vi "Analog Input User Interface.vi"() -> ()   [LabVIEW 2023, in "GUI.lvlib" / "Diagnostic.lvlib"]
uses:
  Diagnostic.lvlib
  Control/Analog Input 6345.ctl
  Control/Analog Input.ctl
  Control/Analog Input 6363.ctl
  HardwareAbstractionLayer_LVOOP/Analog Input/NI Analog Input/NI Analog Input.lvclass
  D:/eDCU LTT/VT LTT Project/Source Code/HardwareAbstractionLayer_LVOOP/Analog Input/AI/AI.lvclass
  HardwareAbstractionLayer_LVOOP/Database/SQL Public VI/Control/DB Options.ctl
  HardwareAbstractionLayer_LVOOP/Main/Class Ref.ctl
  HardwareAbstractionLayer_LVOOP/DMM/DMM.lvclass
  HardwareAbstractionLayer_LVOOP/Function Generator/Function Generator.lvclass
  HardwareAbstractionLayer_LVOOP/Oscilloscope/Oscilloscope.lvclass
  HardwareAbstractionLayer_LVOOP/PowerSupply/PowerSupply.lvclass
  HardwareAbstractionLayer_LVOOP/Teststand/Teststand.lvclass
  HardwareAbstractionLayer_LVOOP/Analog Output/AO/AO.lvclass
  HardwareAbstractionLayer_LVOOP/Analog Input/AI/AI.lvclass
  HardwareAbstractionLayer_LVOOP/Database/Database.lvclass
  HardwareAbstractionLayer_LVOOP/Digital Output/DO_class/DO.lvclass
  HardwareAbstractionLayer_LVOOP/Digital Input/DI_class/DI.lvclass
  HardwareAbstractionLayer_LVOOP/PWM Output/PWM Output_class/PWM Output.lvclass
  HardwareAbstractionLayer_LVOOP/PWM Input/PWM Input_class/PWM Input.lvclass
  HardwareAbstractionLayer_LVOOP/NI Switch/NISwitch_class/NISwitch.lvclass
  HardwareAbstractionLayer_LVOOP/Modbus/Modbus_class/Modbus.lvclass
  HardwareAbstractionLayer_LVOOP/CAN/CAN Lib/CAN_class/CAN.lvclass
  HardwareAbstractionLayer_LVOOP/Main/Main.lvclass
panel:
  in  "Stop Acquire":bool
  in  "Start Acquire":bool
  out "error out":errorcluster
  in  "error in":errorcluster
  in  "Operation":enum32{"6345-PXI2Slot3", "6363-PXI2Slot2"}(tab)
  out "PXIe - 6345":T1 {"Channel 31" format="%.3g"; "Channel 30" format="%.3g"; "Channel 29" format="%.3g"; "Channel 28" format="%.3g"; "Channel 27" format="%.3g"; "Channel 26" format="%.3g"; "Channel 25" format="%.3g"; "Channel 24" format="%.3g"; "Channel 23" format="%.3g"; "Channel 22" format="%.3g"; "Channel 21" format="%.3g"; "Channel 20" format="%.3g"; "Channel 19" format="%.3g"; "Channel 18" format="%.3g"; "Channel 17" format="%.3g"; "Channel 16" format="%.3g"; "Channel 79" format="%.3g"; "Channel 78" format="%.3g"; "Channel 77" format="%.3g"; "Channel 76" format="%.3g"; "Channel 75" format="%.3g"; "Channel 74" format="%.3g"; "Channel 73" format="%.3g"; "Channel 72" format="%.3g"; "Channel 71" format="%.3g"; "Channel 70" format="%.3g"; "Channel 69" format="%.3g"; "Channel 68" format="%.3g"; "Channel 67" format="%.3g"; "Channel 66" format="%.3g"; "Channel 65" format="%.3g"; "Channel 64" format="%.3g"; "Channel 63" format="%.3g"; "Channel 62" format="%.3g"; "Channel 61" format="%.3g"; "Channel 60" format="%.3g"; "Channel 59" format="%.3g"; "Channel 58" format="%.3g"; "Channel 57" format="%.3g"; "Channel 56" format="%.3g"; "Channel 55" format="%.3g"; "Channel 54" format="%.3g"; "Channel 53" format="%.3g"; "Channel 52" format="%.3g"; "Channel 51" format="%.3g"; "Channel 50" format="%.3g"; "Channel 49" format="%.3g"; "Channel 48" format="%.3g"; "Channel 47" format="%.3g"; "Channel 46" format="%.3g"; "Channel 45" format="%.3g"; "Channel 44" format="%.3g"; "Channel 43" format="%.3g"; "Channel 42" format="%.3g"; "Channel 41" format="%.3g"; "Channel 40" format="%.3g"; "Channel 39" format="%.3g"; "Channel 38" format="%.3g"; "Channel 37" format="%.3g"; "Channel 36" format="%.3g"; "Channel 35" format="%.3g"; "Channel 34" format="%.3g"; "Channel 33" format="%.3g"; "Channel 32" format="%.3g"; "Channel 15" format="%.3g"; "Channel 14" format="%.3g"; "Channel 13" format="%.3g"; "Channel 12" format="%.3g"; "Channel 11" format="%.3g"; "Channel 10" format="%.3g"; "Channel 9" format="%.3g"; "Channel 8" format="%.3g"; "Channel 7" format="%.3g"; "Channel 6" format="%.3g"; "Channel 5" format="%.3g"; "Channel 4" format="%.3g"; "Channel 3" format="%.3g"; "Channel 2" format="%.3g"; "Channel 1" format="%.3g"; "Channel 0" format="%.3g"}
  out "PXIe - 6363":T3 {"Channel 31" format="%.3g"; "Channel 30" format="%.3g"; "Channel 29" format="%.3g"; "Channel 28" format="%.3g"; "Channel 27" format="%.3g"; "Channel 26" format="%.3g"; "Channel 25" format="%.3g"; "Channel 24" format="%.3g"; "Channel 23" format="%.3g"; "Channel 22" format="%.3g"; "Channel 21" format="%.3g"; "Channel 20" format="%.3g"; "Channel 19" format="%.3g"; "Channel 18" format="%.3g"; "Channel 17" format="%.3g"; "Channel 16" format="%.3g"; "Channel 15" format="%.3g"; "Channel 14" format="%.3g"; "Channel 13" format="%.3g"; "Channel 12" format="%.3g"; "Channel 11" format="%.3g"; "Channel 10" format="%.3g"; "Channel 9" format="%.3g"; "Channel 8" format="%.3g"; "Channel 7" format="%.3g"; "Channel 6" format="%.3g"; "Channel 5" format="%.3g"; "Channel 4" format="%.3g"; "Channel 3" format="%.3g"; "Channel 2" format="%.3g"; "Channel 1" format="%.3g"; "Channel 0" format="%.3g"}
  in  "Stop":bool caption="Blank"
  # "Analog Input"
  # "Device:"
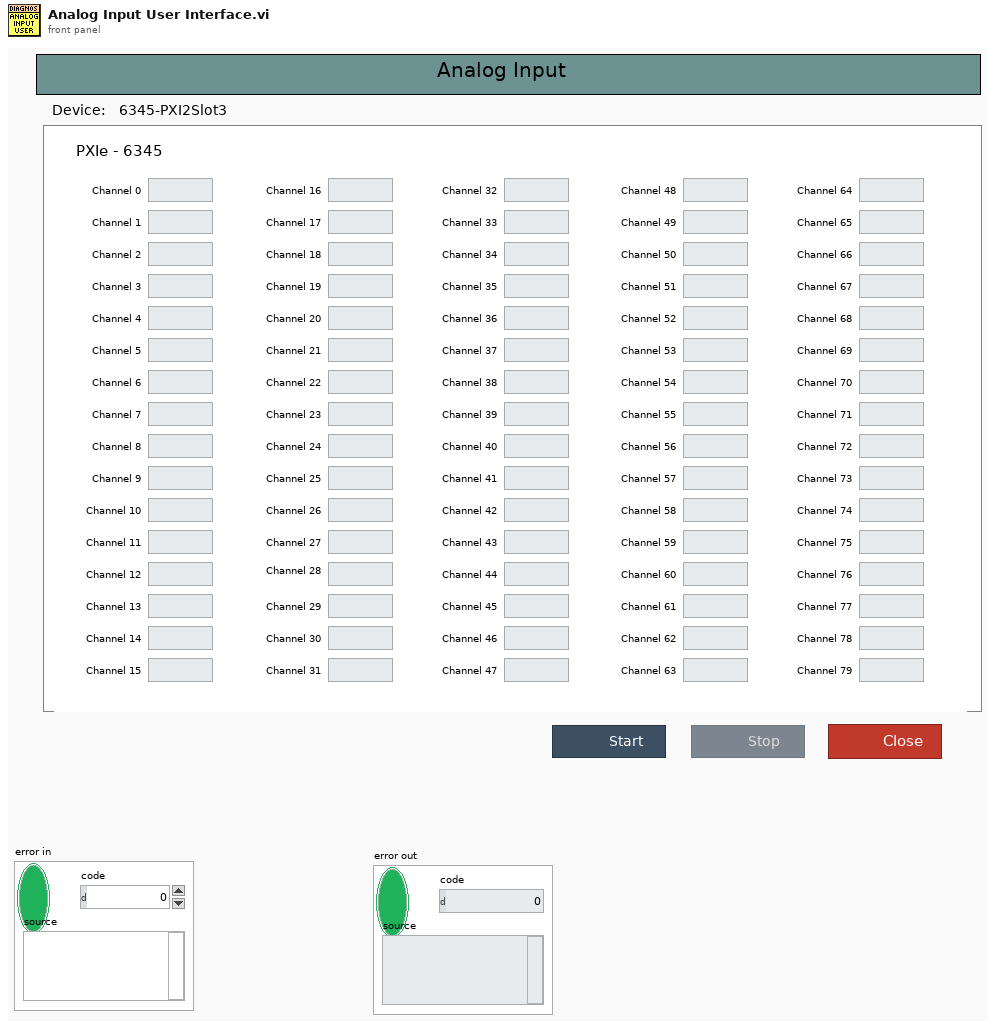
[diagram p1: front panel]
types:
  T1 = typedef "GUI.lvlib/Diagnostic.lvlib/Analog Input 6345.ctl" = cluster{"Channel 0":T2, "Channel 1":T2, "Channel 2":T2, "Channel 3":T2, "Channel 4":T2, "Channel 5":T2, "Channel 6":T2, "Channel 7":T2, "Channel 8":T2, "Channel 9":T2, "Channel 10":T2, "Channel 11":T2, "Channel 12":T2, "Channel 13":T2, "Channel 14":T2, "Channel 15":T2, "Channel 16":T2, "Channel 17":T2, "Channel 18":T2, "Channel 19":T2, "Channel 20":T2, "Channel 21":T2, "Channel 22":T2, "Channel 23":T2, "Channel 24":T2, "Channel 25":T2, "Channel 26":T2, "Channel 27":T2, "Channel 28":T2, "Channel 29":T2, "Channel 30":T2, "Channel 32":T2, "Channel 33":T2, "Channel 34":T2, "Channel 35":T2, "Channel 36":T2, "Channel 37":T2, "Channel 38":T2, "Channel 39":T2, "Channel 40":T2, "Channel 41":T2, "Channel 42":T2, "Channel 43":T2, "Channel 44":T2, "Channel 45":T2, "Channel 46":T2, "Channel 47":T2, "Channel 48":T2, "Channel 49":T2, "Channel 50":T2, "Channel 51":T2, "Channel 52":T2, "Channel 53":T2, "Channel 54":T2, "Channel 55":T2, "Channel 56":T2, "Channel 57":T2, "Channel 58":T2, "Channel 59":T2, "Channel 60":T2, "Channel 61":T2, "Channel 62":T2, "Channel 63":T2, "Channel 64":T2, "Channel 65":T2, "Channel 66":T2, "Channel 67":T2, "Channel 68":T2, "Channel 69":T2, "Channel 70":T2, "Channel 71":T2, "Channel 72":T2, "Channel 73":T2, "Channel 74":T2, "Channel 75":T2, "Channel 76":T2, "Channel 77":T2, "Channel 78":T2, "Channel 79":T2, "Channel 31":T2}
  T2 = typedef "GUI.lvlib/Diagnostic.lvlib/Analog Input.ctl" = dbl
  T3 = typedef "GUI.lvlib/Diagnostic.lvlib/Analog Input 6363.ctl" = cluster{"Channel 0":T2, "Channel 1":T2, "Channel 2":T2, "Channel 3":T2, "Channel 4":T2, "Channel 5":T2, "Channel 6":T2, "Channel 7":T2, "Channel 8":T2, "Channel 9":T2, "Channel 10":T2, "Channel 11":T2, "Channel 12":T2, "Channel 13":T2, "Channel 14":T2, "Channel 15":T2, "Channel 16":T2, "Channel 17":T2, "Channel 18":T2, "Channel 19":T2, "Channel 20":T2, "Channel 21":T2, "Channel 22":T2, "Channel 23":T2, "Channel 24":T2, "Channel 25":T2, "Channel 26":T2, "Channel 27":T2, "Channel 28":T2, "Channel 29":T2, "Channel 30":T2, "Channel 31":T2}
  T4 = typedef "HardwareAbstractionLayer_LVOOP.lvlib/Database.lvclass/DB Options.ctl" = enum16{"Init", "Select Data", "Insert Data", "Update Data", "Delete Data", "Execute Query", "Create Schema", "Create Table", "List Tables", "List Columns", "Close"}
  T5 = typedef "HardwareAbstractionLayer_LVOOP.lvlib/Main.lvclass/Class Ref.ctl" = cluster{"DMM":refnum<class "DMM.lvclass">, "Function Generator":refnum<class "Function Generator.lvclass">, "Oscilloscope":refnum<class "Oscilloscope.lvclass">, "PowerSupply":refnum<class "PowerSupply.lvclass">, "Teststand":refnum<class "Teststand.lvclass">, "AO":refnum<class "AO.lvclass">, "AI":refnum<class "AI.lvclass">, "Database":refnum<class "Database.lvclass">, "AO Waveform Generation":refnum<class "AO.lvclass">, "DO":refnum<class "DO.lvclass">, "DI":refnum<class "DI.lvclass">, "PWM Output":refnum<class "PWM Output.lvclass">, "PWM Input":refnum<class "PWM Input.lvclass">, "RelayOutput":refnum<class "NISwitch.lvclass">, "Modbus":refnum<class "Modbus.lvclass">, "CAN":refnum<class "CAN.lvclass">}
  T6 = enum8{"Enabled", "Disabled", "Disabled and Grayed Out"}
  T7 = cluster{"data[0]":dbl, "data[1]":dbl, "data[2]":dbl, "data[3]":dbl, "data[4]":dbl, "data[5]":dbl, "data[6]":dbl, "data[7]":dbl, "data[8]":dbl, "data[9]":dbl, "data[10]":dbl, "data[11]":dbl, "data[12]":dbl, "data[13]":dbl, "data[14]":dbl, "data[15]":dbl, "data[16]":dbl, "data[17]":dbl, "data[18]":dbl, "data[19]":dbl, "data[20]":dbl, "data[21]":dbl, "data[22]":dbl, "data[23]":dbl, "data[24]":dbl, "data[25]":dbl, "data[26]":dbl, "data[27]":dbl, "data[28]":dbl, "data[29]":dbl, "data[30]":dbl, "data[31]":dbl, "data[32]":dbl, "data[33]":dbl, "data[34]":dbl, "data[35]":dbl, "data[36]":dbl, "data[37]":dbl, "data[38]":dbl, "data[39]":dbl, "data[40]":dbl, "data[41]":dbl, "data[42]":dbl, "data[43]":dbl, "data[44]":dbl, "data[45]":dbl, "data[46]":dbl, "data[47]":dbl, "data[48]":dbl, "data[49]":dbl, "data[50]":dbl, "data[51]":dbl, "data[52]":dbl, "data[53]":dbl, "data[54]":dbl, "data[55]":dbl, "data[56]":dbl, "data[57]":dbl, "data[58]":dbl, "data[59]":dbl, "data[60]":dbl, "data[61]":dbl, "data[62]":dbl, "data[63]":dbl, "data[64]":dbl, "data[65]":dbl, "data[66]":dbl, "data[67]":dbl, "data[68]":dbl, "data[69]":dbl, "data[70]":dbl, "data[71]":dbl, "data[72]":dbl, "data[73]":dbl, "data[74]":dbl, "data[75]":dbl, "data[76]":dbl, "data[77]":dbl, "data[78]":dbl, "data[79]":dbl}
  T8 = cluster{"data[0]":dbl, "data[1]":dbl, "data[2]":dbl, "data[3]":dbl, "data[4]":dbl, "data[5]":dbl, "data[6]":dbl, "data[7]":dbl, "data[8]":dbl, "data[9]":dbl, "data[10]":dbl, "data[11]":dbl, "data[12]":dbl, "data[13]":dbl, "data[14]":dbl, "data[15]":dbl, "data[16]":dbl, "data[17]":dbl, "data[18]":dbl, "data[19]":dbl, "data[20]":dbl, "data[21]":dbl, "data[22]":dbl, "data[23]":dbl, "data[24]":dbl, "data[25]":dbl, "data[26]":dbl, "data[27]":dbl, "data[28]":dbl, "data[29]":dbl, "data[30]":dbl, "data[31]":dbl}
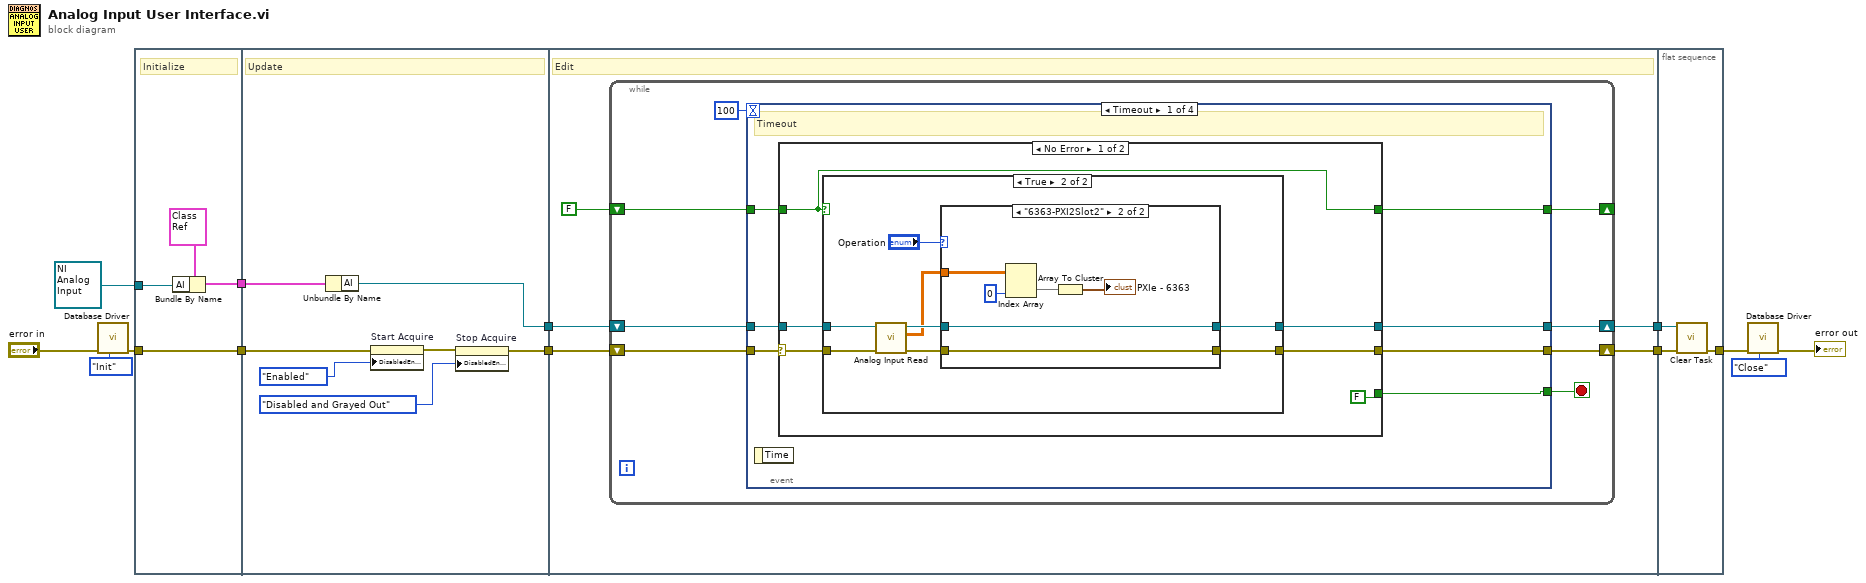
[diagram p0: block diagram]
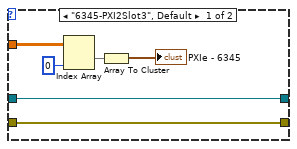
[diagram p3: hidden frame]
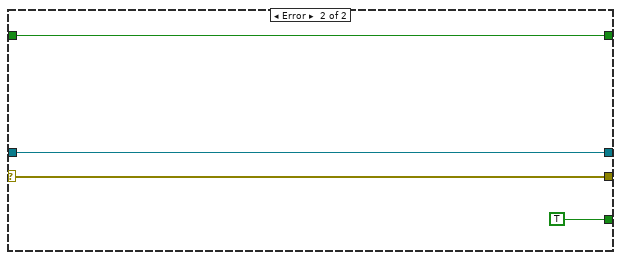
[diagram p4: hidden frame]
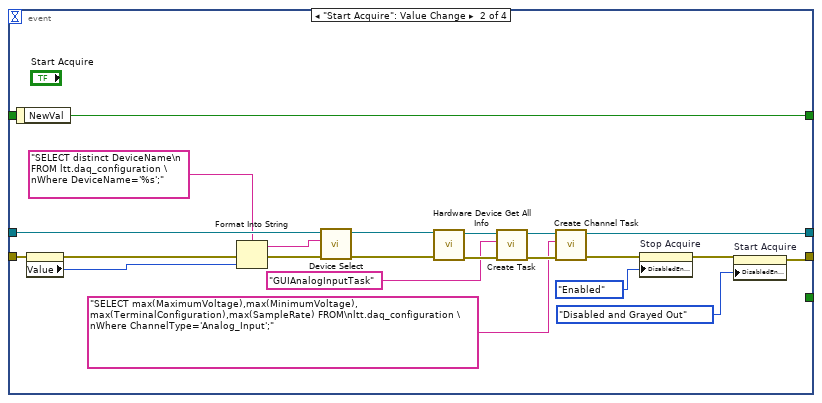
[diagram p5: hidden frame]
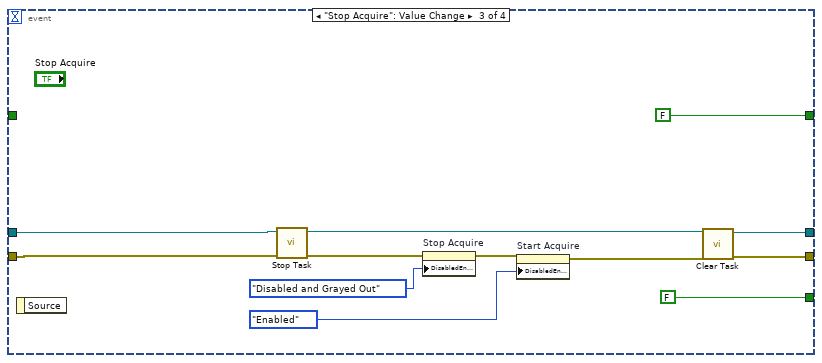
[diagram p6: hidden frame]
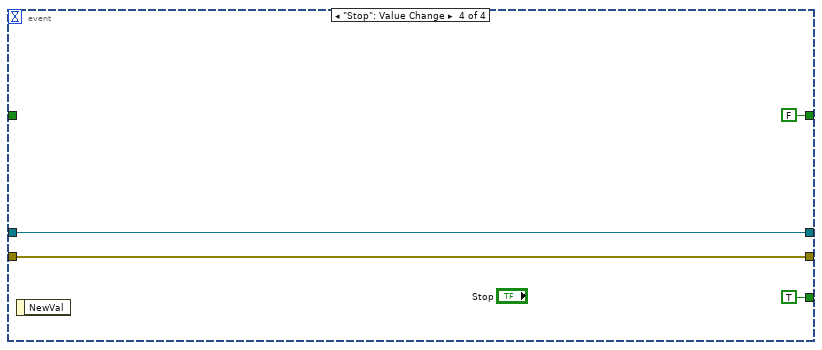
[diagram p7: hidden frame]
diagram:
  n1 = call "Database Driver.vi"("Options"=DB_Options."Init", "error in"="error in") -> ("error out"=w3:errorcluster)  [unwired: 6 in, 3 out]
  n2 = flat-sequence {
    tunnel: [w17] -> w11
    tunnel: w3 -> [w17]
    tunnel: refnum<class "NI Analog Input.lvclass"> refnum ("HardwareAbstractionLayer_LVOOP.lvlib:NI Analog Input.lvclass") -> [w15]
    tunnel: [w14] -> w10
    tunnel: w11 -> [w21]
    tunnel: [w20] -> w9
    tunnel: w10 -> [w24]
    tunnel: [w23] -> w8
    tunnel: w9 -> [w29]
    tunnel: w8 -> [w27]
    tunnel: [w28] -> w7
    tunnel: [w26] -> w6
    tunnel: [w115] -> w1
    tunnel: w7 -> [w116]
    tunnel: w6 -> [w117]
    frame #0 {
      # "Initialize"
      n3 = Bundle By Name(cluster=T5 {"DMM"=refnum, "Function Generator"=refnum, "Oscilloscope"=refnum, "PowerSupply"=refnum, "Teststand"=refnum, "AO"=refnum, "AI"=refnum, "Database"=refnum, "AO Waveform Generation"=refnum, "DO"=refnum, "DI"=refnum, "PWM Output"=refnum, "PWM Input"=refnum, "RelayOutput"=refnum, "Modbus"=refnum, "CAN"=refnum} ("Class Cluster"), "AI"=w15) -> (w14:T5)
    }
    frame #1 {
      # "Update"
      n4 = Unbundle By Name(w24) -> ("AI"=w23:refnum<class "AI.lvclass">)
      n5 = property on="Start Acquire" class="Bool"(error in=w21, "DisabledEnum"=T6."Enabled" ("Disabled")) -> (error out=w22:errorcluster)  [unwired: 1 in, 1 out]
      n6 = property on="Stop Acquire" class="Bool"(error in=w22, "DisabledEnum"=T6."Disabled and Grayed Out" ("Disabled")) -> (error out=w20:errorcluster)  [unwired: 1 in, 1 out]
    }
    frame #2 {
      # "Edit"
      n7 = while {
        shift-right: [w32] -> w26
        shift-left: w27 -> [w33]
        shift-right: [w34] -> w28
        shift-left: w29 -> [w35]
        shift-right: [w31] -> _
        shift-left: FALSE ("NewVal") -> [w30]
        stop <- w36 stop-if-true
        n8 = event shown="[0] Timeout" {
          selector: _ -> [_ _ _ _]
          dyn-events: _ -> [_ _ _ _]
          timeout: 100 -> [_ _ _ _]
          tunnel: [w40 _ FALSE ("Stop") TRUE ("Stop")] -> w36
          tunnel: w35 -> [w44 w95 w109 w113]
          tunnel: [w43 w79 w101 w113] -> w34
          tunnel: w33 -> [w42 w98 w110 w114]
          tunnel: [w41 w83 w99 w114] -> w32
          tunnel: [w38 w82 FALSE ("NewVal") FALSE ("NewVal")] -> w31
          tunnel: w30 -> [w39 _ _ _]
          event Timeout {
            # "Timeout"
            n9 = event-data() -> ()  [unwired: 1 in, 1 out]
            n10 = case shown="No Error" w44 {
              selector: w44 -> [w48 w76]
              tunnel: [w50 w76] -> w43
              tunnel: w42 -> [w47 w75]
              tunnel: [w49 w75] -> w41
              tunnel: [FALSE ("Stop") TRUE ("Stop")] -> w40
              tunnel: w39 -> [w45 w73]
              tunnel: [w45 w73] -> w38
              frame No Error {
                n11 = case shown="True" w45 {
                  tunnel: [w51 w60] -> w50
                  tunnel: [w52 w58] -> w49
                  tunnel: w48 -> [w51 w57]
                  tunnel: w47 -> [w52 w55]
                  frame False {
                  }
                  frame True {
                    n12 = call-dynamic "Analog Input Read.vi"("error in (no error)"=w57, "AI in"=w55) -> ("error out"=w56:errorcluster, "data"=w53:dbl[][], "AI out"=w54:refnum<class "AI.lvclass">)  [unwired: 7 in]
                    n13 = case shown="\"6363-PXI2Slot2\"" "Operation" {
                      tunnel: w56 -> [w63 w68]
                      tunnel: [w63 w68] -> w60
                      tunnel: w54 -> [w64 w69]
                      tunnel: [w64 w69] -> w58
                      tunnel: w53 -> [w62 w70]
                      frame "6345-PXI2Slot3", Default {
                        n14 = Index Array(array=w62, index (col)=0 ("disabled index (col)")) -> (element=w66:dbl[])  [unwired: 1 in]
                        n15 = Array To Cluster(array=w66) -> (cluster=→"PXIe - 6345":T7)
                      }
                      frame "6363-PXI2Slot2" {
                        n16 = Index Array(array=w70, index (col)=0 ("disabled index (col)")) -> (element=w71:dbl[])  [unwired: 1 in]
                        n17 = Array To Cluster(array=w71) -> (cluster=→"PXIe - 6363":T8)
                      }
                    }
                  }
                }
              }
              frame Error {
              }
            }
          }
          event "Start Acquire": Value Change {
            n18 = event-data() -> ("NewVal"=w82:bool)  [unwired: 1 in]
            n19 = property on="Operation" class="TabCtl (strict)"(error in=w95) -> (error out=w96:errorcluster, "Value"=w97:enum32{"6345-PXI2Slot3", "6363-PXI2Slot2"})  [unwired: 1 in, 1 out]
            n20 = Format Into String(format string="SELECT distinct DeviceName\n FROM ltt.daq_configuration \nWhere DeviceName='%s';" ("SQL query"), error in=w96, w97) -> (resulting string=w92:string, error out=w94:errorcluster)  [unwired: 1 in]
            n21 = call-dynamic "Device Select.vi"("error in (no error)"=w94, "SQL query"=w92, "AI in"=w98) -> ("error out"=w84:errorcluster, "AI out"=w85:refnum<class "AI.lvclass">)  [unwired: 7 in]
            n22 = call-dynamic "Hardware Device Get All Info.vi"("error in (no error)"=w84, "AI in"=w85) -> ("error out"=w89:errorcluster, "AI out"=w88:refnum<class "AI.lvclass">)  [unwired: 8 in]
            n23 = call-dynamic "Create Task.vi"("error in (no error)"=w89, "Task name"="GUIAnalogInputTask", "AI in"=w88) -> ("error out"=w90:errorcluster, "AI out"=w91:refnum<class "AI.lvclass">)  [unwired: 7 in]
            n24 = call-dynamic "Create Channel Task.vi"("error in (no error)"=w90, "SQL query"="SELECT max(MaximumVoltage),max(MinimumVoltage), max(TerminalConfiguration),max(SampleRate) FROM\nltt.daq_configuration \nWhere ChannelType='Analog_Input';", "AI in"=w91) -> ("error out"=w81:errorcluster, "AI out"=w83:refnum<class "AI.lvclass">)  [unwired: 7 in]
            n25 = property on="Stop Acquire" class="Bool"(error in=w81, "DisabledEnum"=T6."Enabled" ("Disabled")) -> (error out=w80:errorcluster)  [unwired: 1 in, 1 out]
            n26 = property on="Start Acquire" class="Bool"(error in=w80, "DisabledEnum"=T6."Disabled and Grayed Out" ("Disabled")) -> (error out=w79:errorcluster)  [unwired: 1 in, 1 out]
          }
          event "Stop Acquire": Value Change {
            n27 = event-data() -> ()  [unwired: 1 in, 1 out]
            n28 = call-dynamic "Stop Task.vi"("error in (no error)"=w109, "AI in"=w110) -> ("error out"=w103:errorcluster, "AI out"=w100:refnum<class "AI.lvclass">)  [unwired: 8 in]
            n29 = property on="Stop Acquire" class="Bool"(error in=w103, "DisabledEnum"=T6."Disabled and Grayed Out" ("Disabled")) -> (error out=w106:errorcluster)  [unwired: 1 in, 1 out]
            n30 = property on="Start Acquire" class="Bool"(error in=w106, "DisabledEnum"=T6."Enabled" ("Disabled")) -> (error out=w102:errorcluster)  [unwired: 1 in, 1 out]
            n31 = call-dynamic "Clear Task.vi"("error in (no error)"=w102, "AI in"=w100) -> ("error out"=w101:errorcluster, "AI out"=w99:refnum<class "AI.lvclass">)  [unwired: 8 in]
          }
          event "Stop": Value Change {
            n32 = event-data() -> ()  [unwired: 1 in, 1 out]
          }
        }
      }
    }
    frame #3 {
      n33 = call-dynamic "Clear Task.vi"("error in (no error)"=w116, "AI in"=w117) -> ("error out"=w115:errorcluster)  [unwired: 8 in, 1 out]
    }
  }
  n34 = call "Database Driver.vi"("Options"=DB_Options."Close", "error in"=w1) -> ("error out"=→"error out":errorcluster)  [unwired: 6 in, 3 out]
